vi "getUnitId.vi"(8 "error in (no error)":errorcluster) -> (0 "error out":errorcluster, 3 "UnitId":T1)   [LabVIEW 2010, in "TPVG_DLL.lvlib"]
doc: "------------------------------------------\nAuthor: Dang Lam\nEmail: danglamtd@gmail.com"
uses:
  TPVG_DLL.lvlib
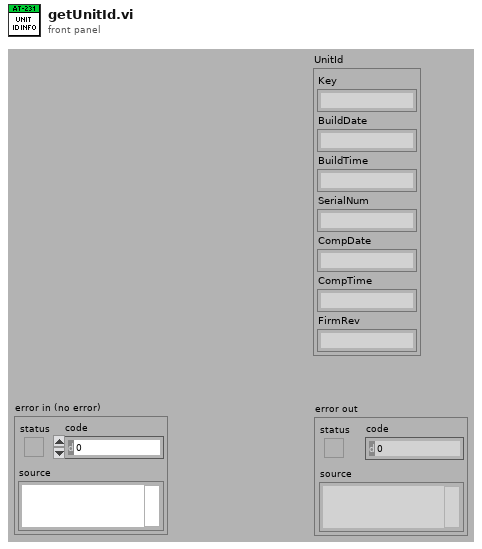
[diagram p1: front panel]
types:
  T1 = cluster{"Key":string, "BuildDate":string, "BuildTime":string, "SerialNum":string, "CompDate":string, "CompTime":string, "FirmRev":string}
  T2 = cluster{string, string, string, string, string, string, string}
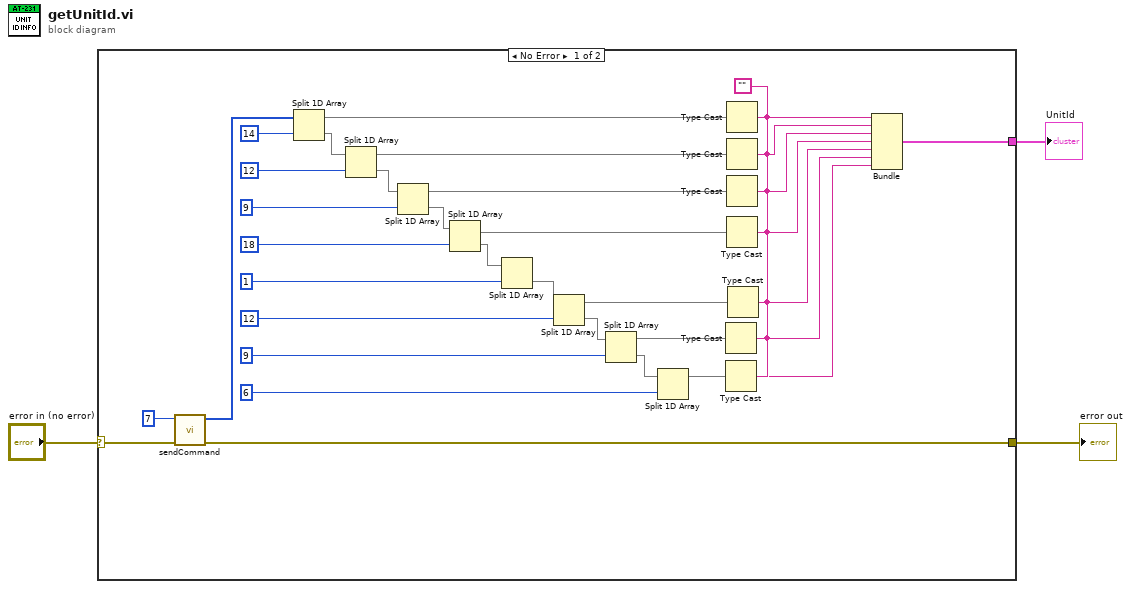
[diagram p0: block diagram]
diagram:
  n1 = case shown="No Error" "error in (no error)" {
    selector: "error in (no error)" -> [w38 w39]
    tunnel: [w36 w39] -> w2
    tunnel: [w4 _] -> w1
    frame No Error {
      w14 = ""
      n2 = call "sendCommand.vi"("error in (no error)"=w38, "Command ID"=u16 7) -> ("error out"=w36:errorcluster, "Data out"=w35:u8[])  [unwired: 8 in]
      n3 = Split 1D Array(array=w35, index=14) -> (first subarray=w33:u8[], second subarray=w32:u8[])
      n4 = Split 1D Array(array=w32, index=12) -> (first subarray=w30:u8[], second subarray=w29:u8[])
      n5 = Split 1D Array(array=w29, index=9) -> (first subarray=w27:u8[], second subarray=w26:u8[])
      n6 = Split 1D Array(array=w26, index=18) -> (first subarray=w24:u8[], second subarray=w23:u8[])
      n7 = Split 1D Array(array=w23, index=1) -> (second subarray=w21:u8[])  [unwired: 1 out]
      n8 = Split 1D Array(array=w21, index=12) -> (first subarray=w15:u8[], second subarray=w19:u8[])
      n9 = Split 1D Array(array=w19, index=9) -> (first subarray=w13:u8[], second subarray=w17:u8[])
      n10 = Split 1D Array(array=w17, index=6) -> (first subarray=w12:u8[])  [unwired: 1 out]
      n11 = Type Cast(type=w14, x=w13) -> (*(type *) &x=w6:string)
      n12 = Type Cast(type=w14, x=w12) -> (*(type *) &x=w5:string)
      n13 = Type Cast(type=w14, x=w33) -> (*(type *) &x=w11:string)
      n14 = Type Cast(type=w14, x=w30) -> (*(type *) &x=w10:string)
      n15 = Type Cast(type=w14, x=w27) -> (*(type *) &x=w9:string)
      n16 = Type Cast(type=w14, x=w24) -> (*(type *) &x=w8:string)
      n17 = Type Cast(type=w14, x=w15) -> (*(type *) &x=w7:string)
      n18 = Bundle(w11, w10, w9, w8, w7, w6, w5) -> (w4:T2)  [unwired: 1 in]
    }
    frame Error {
    }
  }
  "error out" <- w2
  "UnitId" <- w1
